vi "targetRead.vi"() -> ()   [LabVIEW 2017]
panel:
  out "error IO":errorcluster
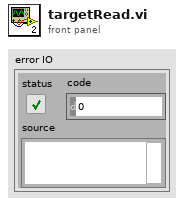
[diagram p1: front panel]
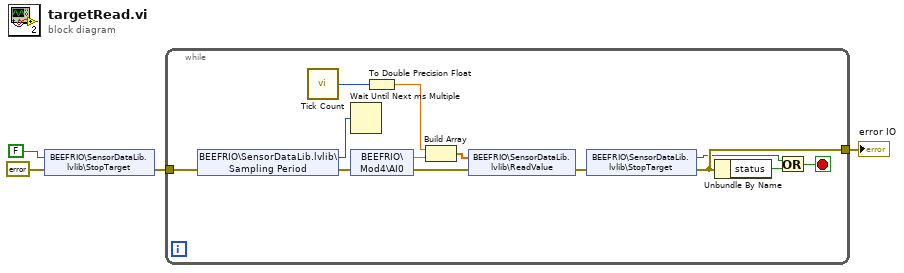
[diagram p0: block diagram]
diagram:
  n1 = shared-variable "BEEFRIO\\SensorDataLib.lvlib\\StopTarget"(FALSE ("StopTarget"), error in=errorcluster {"status"=FALSE, "code"=0, "source"=""} ("error in (no error)")) -> (error out=w4:errorcluster)
  n2 = while {
    tunnel: w4 -> [w16]
    tunnel: [w9] -> w1
    stop <- w6 stop-if-true
    n3 = shared-variable "BEEFRIO\\SensorDataLib.lvlib\\Sampling Period"(error in=w16) -> (w17:u32, error out=w11:errorcluster)
    n4 = call "Tick Count"() -> ("Tick Count(uSec)"=w15:u32)
    n5 = Wait Until Next ms Multiple(millisecond multiple=w17) -> ()  [unwired: 1 out]
    n6 = shared-variable "BEEFRIO\\Mod4\\AI0"(error in=w11) -> (w13:dbl, error out=w5:errorcluster)
    n7 = To Double Precision Float(number=w15) -> (double precision float=w14:dbl)
    n8 = Build Array(w14, w13) -> (w12:dbl[])
    n9 = shared-variable "BEEFRIO\\SensorDataLib.lvlib\\ReadValue"(w12, error in=w5) -> (error out=w10:errorcluster)
    n10 = shared-variable "BEEFRIO\\SensorDataLib.lvlib\\StopTarget"(error in=w10) -> (w7:bool, error out=w9:errorcluster)
    n11 = Unbundle By Name(w9) -> ("status"=w8:bool)
    n12 = Or(x=w7, y=w8) -> (x .or. y?=w6:bool)
  }
  "error IO" <- w1
